vi "Robot Global Data.vi"() -> ()   [LabVIEW 2015]
doc: "This global VI can contain as many global variables as you need. Place a control on the panel, give it a good name. To read or write to it from a VI, drag the icon to the diagram of that VI. You can also drag from the project. Click on the node to change which global you access. You shouldn't have multiple locations writing to a global or it will cause a race-condition."
uses:
  <vilib>/Rock Robotics/WPI/DriverStation/WPI_DriverStationRobotMode2.ctl
  <vilib>/Rock Robotics/WPI/Camera/WPI_CameraImageSize.ctl
panel:
  in  "LowOut":bool
  in  "SlowRotate":bool
  out "ManipPosition":dbl
  in  "ManipSetPoint":dbl
  out "ShootStart":u32
  in  "CataCase":u16(ring) items=["0", "1"]
  in  "GyroAngle":dbl
  in  "GyroReset":bool
  in  "AngleLock":bool
  in  "image size":T1=enum."320x240"
  in  "Enable Vision":bool
  out "RightInches":dbl
  out "LeftInches":dbl
  in  "ResetEncoders":bool
  in  "DrivingPID?":bool
  in  "Autonomous?":bool
  out "AxisY":dbl
  out "AxisX":dbl
  in  "CataUp":bool
  in  "ClimbMechUp":bool
  in  "DownClimb":bool
  in  "LiftClimb":bool
  in  "IntakeOUT":bool
  in  "IntakeIN":bool
  in  "Catapult":bool
  in  "Robot Mode":T2
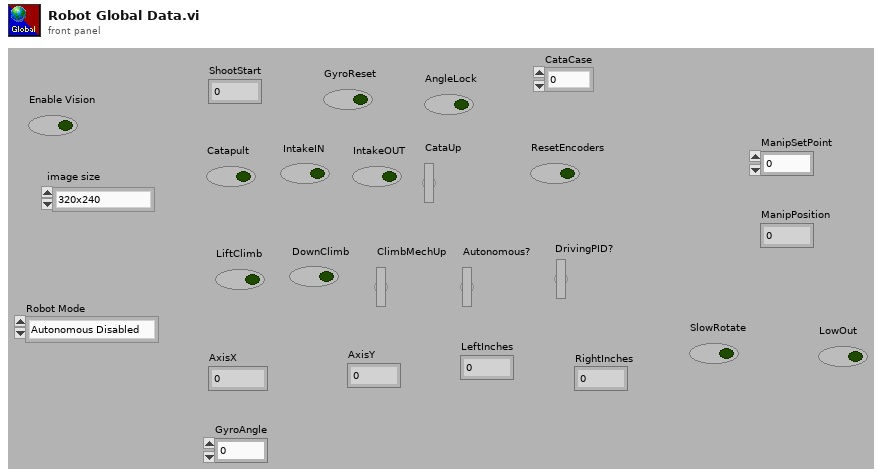
[diagram p1: front panel]
types:
  T1 = typedef "WPI_CameraImageSize.ctl" = enum16{"640x480", "320x240", "160x120", "Custom"}
  T2 = typedef "WPI_DriverStationRobotMode2.ctl" = enum16{"Autonomous Disabled", "Autonomous Enabled", "Teleop Disabled", "Teleop Enabled", "Disconnected", "Finish", "Test Disabled", "Test Enabled", "Emergency Stopped"}
diagram:
